vi "run.vi"(8 "error in (no error)":errorcluster, 11 "CameraManager in":refnum<class "CameraManager.lvclass">) -> (0 "error out":errorcluster, 3 "CameraManager out":refnum<class "CameraManager.lvclass">)   [LabVIEW 2011, in "iManagement.lvlib" / "CameraManager.lvclass"]
uses:
  CameraManager.lvclass
  CameraManager.lvclass/CameraManager.ctl
  Hal/Channels/Camera/CameraController.lvclass
  Tools/Filing/FileSystem/FileSystem.lvclass
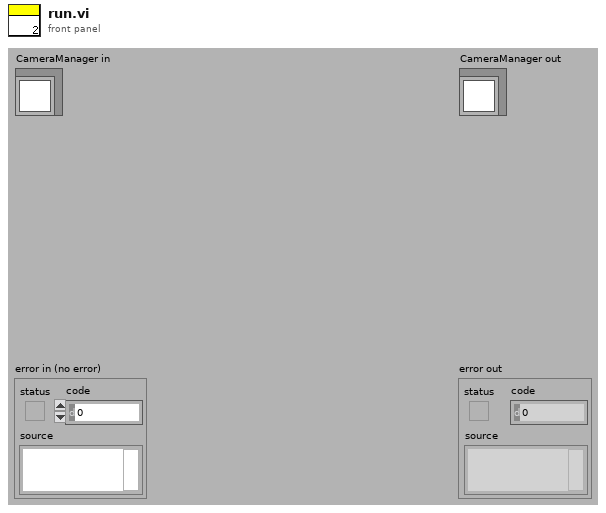
[diagram p1: front panel]
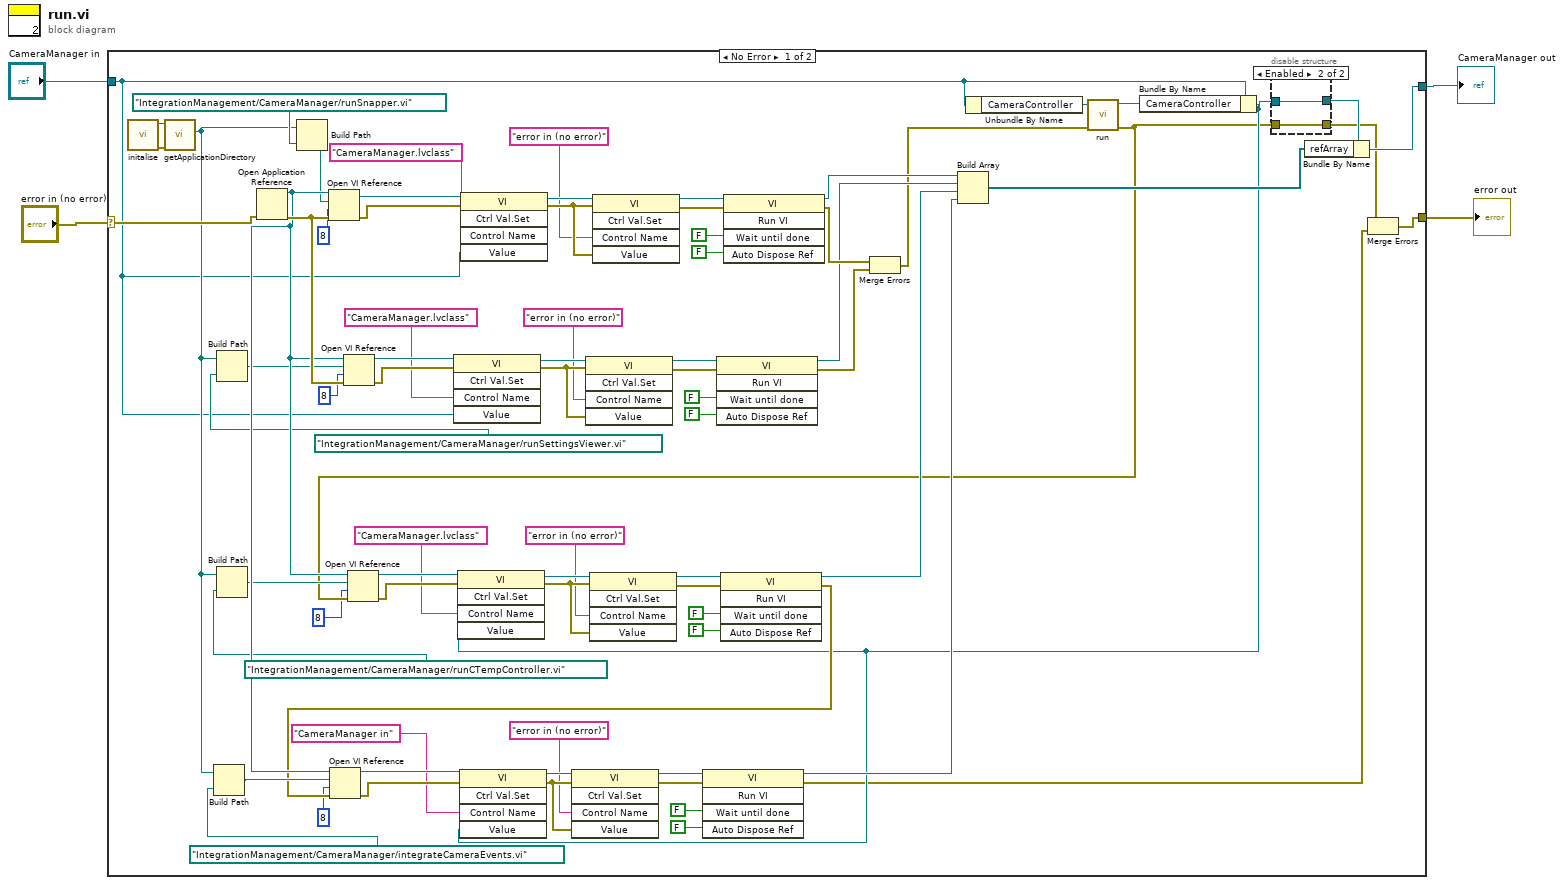
[diagram p0: block diagram]
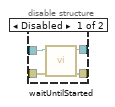
[diagram p2: hidden frame]
diagram:
  n1 = case shown="No Error" "error in (no error)" {
    selector: "error in (no error)" -> [w81 w89]
    tunnel: [w10 w89] -> w3
    tunnel: [w15 w88] -> w1
    tunnel: "CameraManager in" -> [w20 w88]
    frame No Error {
      n2 = call "initalise.vi"() -> ("error out"=w33:errorcluster, "FileSystem out"=w34:refnum<class "FileSystem.lvclass">)  [unwired: 10 in]
      n3 = call-dynamic "getApplicationDirectory.vi"("error in (no error)"=w33, "FileSystem.lvclass in"=w34) -> ("ApplicationDirectory"=w26:path)  [unwired: 7 in, 2 out]
      n4 = Build Path(base path=w26, name or relative path=path "IntegrationManagement/CameraManager/integrateCameraEvents.vi" ("vi path")) -> (appended path=w25:path)
      n5 = Build Path(base path=w26, name or relative path=path "IntegrationManagement/CameraManager/runSettingsViewer.vi" ("vi path")) -> (appended path=w29:path)
      n6 = Build Path(base path=w26, name or relative path=path "IntegrationManagement/CameraManager/runCTempController.vi" ("vi path")) -> (appended path=w27:path)
      n7 = Open Application Reference(8:w81) -> (0:w38:errorcluster, 3:w37:refnum<vi>)  [unwired: 3 in]
      n8 = Build Path(base path=w26, name or relative path=path "IntegrationManagement/CameraManager/runSnapper.vi" ("vi path")) -> (appended path=w31:path)
      n9 = Open VI Reference(application reference (local)=w37, vi path=w31, options=8, error in (no error)=w38) -> (vi reference=w80:refnum<vi>, error out=w79:errorcluster)  [unwired: 2 in]
      n10 = Open VI Reference(application reference (local)=w37, vi path=w29, options=8, error in (no error)=w38) -> (vi reference=w62:refnum<vi>, error out=w63:errorcluster)  [unwired: 2 in]
      n11 = invoke class="VI" method="Ctrl Val.Set"(reference=w62, error in=w63, "Control Name"="CameraManager.lvclass", "Value"=w20) -> (reference out=w69:refnum<vi>, error out=w68:errorcluster)  [unwired: 1 in, 3 out]
      n12 = invoke class="VI" method="Ctrl Val.Set"(reference=w80, error in=w79, "Control Name"="CameraManager.lvclass", "Value"=w20) -> (reference out=w78:refnum<vi>, error out=w77:errorcluster)  [unwired: 1 in, 3 out]
      n13 = invoke class="VI" method="Ctrl Val.Set"(reference=w69, error in=w68, "Control Name"="error in (no error)", "Value"=w68) -> (reference out=w67:refnum<vi>, error out=w66:errorcluster)  [unwired: 1 in, 3 out]
      n14 = invoke class="VI" method="Ctrl Val.Set"(reference=w78, error in=w77, "Control Name"="error in (no error)", "Value"=w77) -> (reference out=w75:refnum<vi>, error out=w74:errorcluster)  [unwired: 1 in, 3 out]
      n15 = invoke class="VI" method="Run VI"(reference=w67, error in=w66, "Wait until done"=FALSE, "Auto Dispose Ref"=FALSE) -> (reference out=w58:refnum<vi>, error out=w70:errorcluster)  [unwired: 1 in, 3 out]
      n16 = invoke class="VI" method="Run VI"(reference=w75, error in=w74, "Wait until done"=FALSE, "Auto Dispose Ref"=FALSE) -> (reference out=w59:refnum<vi>, error out=w71:errorcluster)  [unwired: 1 in, 3 out]
      n17 = Merge Errors(w71, w70) -> (w21:errorcluster)
      n18 = Unbundle By Name(w20) -> ("CameraController"=w23:refnum<class "CameraController.lvclass">)
      n19 = call-dynamic "run.vi"("error in (no error)"=w21, "CameraController in"=w23) -> ("error out"=w6:errorcluster, "CameraController out"=w22:refnum<class "CameraController.lvclass">)  [unwired: 7 in, 1 out]
      n20 = Open VI Reference(application reference (local)=w37, vi path=w27, options=8, error in (no error)=w6) -> (vi reference=w40:refnum<vi>, error out=w41:errorcluster)  [unwired: 2 in]
      n21 = Bundle By Name(cluster=w20, "CameraController"=w22) -> (w14:refnum<class "CameraManager.lvclass">)
      n22 = invoke class="VI" method="Ctrl Val.Set"(reference=w40, error in=w41, "Control Name"="CameraManager.lvclass", "Value"=w14) -> (reference out=w47:refnum<vi>, error out=w46:errorcluster)  [unwired: 1 in, 3 out]
      n23 = invoke class="VI" method="Ctrl Val.Set"(reference=w47, error in=w46, "Control Name"="error in (no error)", "Value"=w46) -> (reference out=w45:refnum<vi>, error out=w44:errorcluster)  [unwired: 1 in, 3 out]
      n24 = invoke class="VI" method="Run VI"(reference=w45, error in=w44, "Wait until done"=FALSE, "Auto Dispose Ref"=FALSE) -> (reference out=w19:refnum<vi>, error out=w18:errorcluster)  [unwired: 1 in, 3 out]
      n25 = Open VI Reference(application reference (local)=w37, vi path=w25, options=8, error in (no error)=w18) -> (vi reference=w50:refnum<vi>, error out=w51:errorcluster)  [unwired: 2 in]
      n26 = invoke class="VI" method="Ctrl Val.Set"(reference=w50, error in=w51, "Control Name"="CameraManager in", "Value"=w14) -> (reference out=w57:refnum<vi>, error out=w56:errorcluster)  [unwired: 1 in, 3 out]
      n27 = invoke class="VI" method="Ctrl Val.Set"(reference=w57, error in=w56, "Control Name"="error in (no error)", "Value"=w56) -> (reference out=w55:refnum<vi>, error out=w54:errorcluster)  [unwired: 1 in, 3 out]
      n28 = invoke class="VI" method="Run VI"(reference=w55, error in=w54, "Wait until done"=FALSE, "Auto Dispose Ref"=FALSE) -> (reference out=w16:refnum<vi>, error out=w11:errorcluster)  [unwired: 1 in, 3 out]
      n29 = Build Array(w59, w58, w19, w16) -> (w17:refnum<vi>[])
      n30 = disable-structure shown="Enabled" {
        disable-tunnel: w14 -> [w85 w87]
        disable-tunnel: [w84 w87] -> w13
        disable-tunnel: [w83 w86] -> w12
        disable-tunnel: w6 -> [w82 w86]
        frame Disabled {
          n31 = call "waitUntilStarted.vi"("error in (no error)"=w82, "CameraManager in"=w85) -> ("error out"=w83:errorcluster, "CameraManager out"=w84:refnum<class "CameraManager.lvclass">)  [unwired: 8 in]
        }
        frame Enabled {
        }
      }
      n32 = Bundle By Name(cluster=w13, "refArray"=w17) -> (w15:refnum<class "CameraManager.lvclass">)
      n33 = Merge Errors(w12, w11) -> (w10:errorcluster)
    }
    frame Error {
    }
  }
  "error out" <- w3
  "CameraManager out" <- w1
